vi "1st.vi"() -> ()   [LabVIEW 2016]
uses:
  <vilib>/Analysis/Matrix/Datatypes/RealMatrix.ctl
  <vilib>/Analysis/Matrix/Numeric/Conversions/Array To Matrix - RA.vi
  <vilib>/Analysis/Matrix/Numeric/Multiply/Multiply - RM,RM.vi
  <vilib>/Analysis/baseanly.llb/Real Inverse Matrix.vi
  <vilib>/Analysis/Matrix/Numeric/Conversions/Matrix To Array - RM.vi
  <vilib>/Analysis/Matrix/NI_Matrix.lvlib
  <vilib>/Analysis/NI_AALBase.lvlib
panel:
  out "r":dbl[](array[numeric])
  out "theta":dbl[](array[numeric])
  out "b":dbl[](array[numeric])
  out "a":dbl[](array[numeric])
  out "Real 2D Array":dbl[][](array[numeric])
  out "Final magnitude":T1
  in  "stop":bool
  out "Inverse Matrix":T1
  out "S(t)* X":T1
  in  "S":T1
  out "Matrix X":T1
  out "Array X":dbl[](array[numeric])
  in  "samples":dbl
  in  "Magnitude":dbl
  in  "Phase":dbl
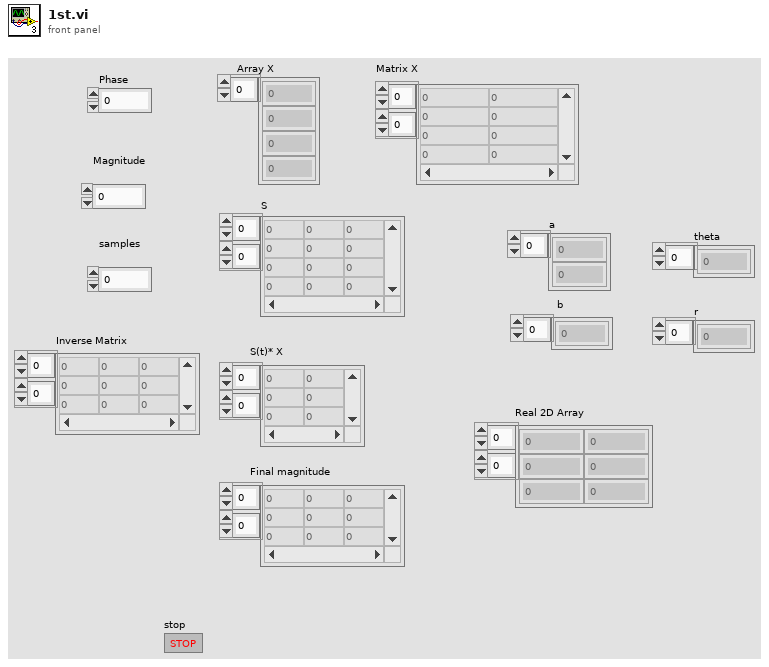
[diagram p1: front panel]
types:
  T1 = typedef "NI_Matrix.lvlib/RealMatrix.ctl" = dbl[][]
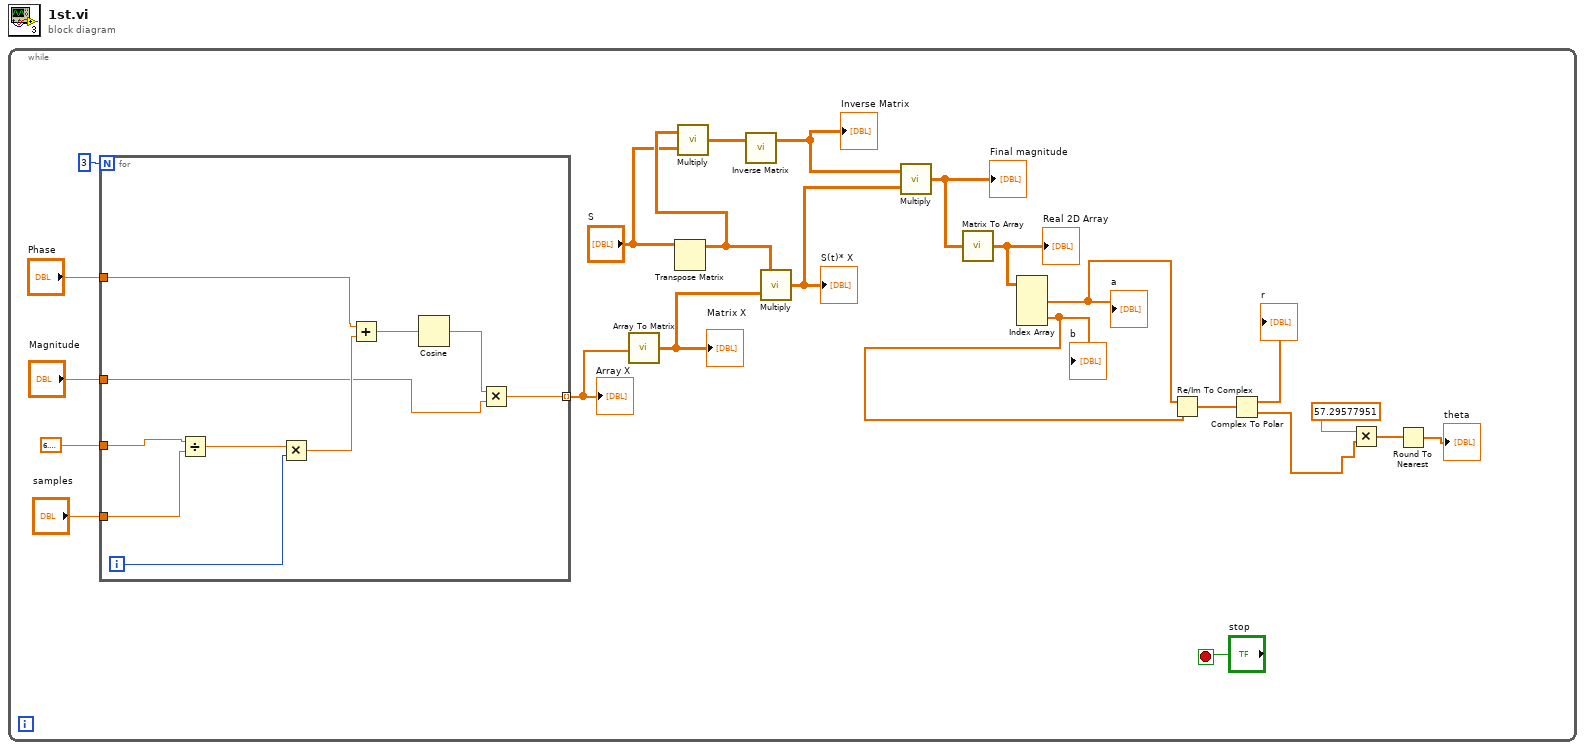
[diagram p0: block diagram]
diagram:
  n1 = while {
    stop <- "stop" stop-if-true
    n2 = for {
      N: 3 -> [_]
      tunnel: 6.283185307179586 -> [w33]
      tunnel: "samples" -> [w32]
      tunnel: "Phase" -> [w28]
      tunnel: "Magnitude" -> [w26]
      tunnel: [w25] -> w18 mode=indexing
      i -> [w30]
      n3 = Divide(x=w33, y=w32) -> (x/y=w31:dbl)
      n4 = Multiply(x=w31, y=w30) -> (x*y=w29:dbl)
      n5 = Add(x=w28, y=w29) -> (x+y=w27:dbl)
      n6 = Cosine(x=w27) -> (cos(x)=w24:dbl)
      n7 = Multiply(x=w24, y=w26) -> (x*y=w25:dbl)
    }
    "Array X" <- w18
    n8 = call-poly <vilib>:"Array To Matrix.vi"("Real 1D Array"=w18) -> ("Real Matrix (Column Vector)"=w17:T1)
    "Matrix X" <- w17
    n9 = Transpose Matrix(1:"S") -> (0:w14:T1)
    n10 = call-poly <vilib>:"Multiply.vi"("Real Matrix B"="S", "Real Matrix A"=w14) -> ("A * B"=w16:T1)
    n11 = call-poly <vilib>:"Inverse Matrix.vi"("Input Matrix"=w16) -> ("Inverse Matrix"=w13:T1)  [unwired: 1 in, 1 out]
    "Inverse Matrix" <- w13
    n12 = call-poly <vilib>:"Multiply.vi"("Real Matrix B"=w17, "Real Matrix A"=w14) -> ("A * B"=w12:T1)
    "S(t)* X" <- w12
    n13 = call-poly <vilib>:"Multiply.vi"("Real Matrix B"=w12, "Real Matrix A"=w13) -> ("A * B"=w11:T1)
    "Final magnitude" <- w11
    n14 = call-poly <vilib>:"Matrix To Array.vi"("Real Matrix"=w11) -> ("Real 2D Array"=w10:dbl[][])
    "Real 2D Array" <- w10
    n15 = Index Array(array=w10) -> (element #1=w9:dbl[], element #2=w8:dbl[])  [unwired: 4 in]
    "a" <- w9
    "b" <- w8
    n16 = Re/Im To Complex(1:w8, 2:w9) -> (0:w7:cdb[])
    n17 = Complex To Polar(r * e^(i*theta)=w7) -> (r=→"r":dbl[], theta=w4:dbl[])
    n18 = Multiply(x=57.29577951, y=w4) -> (x*y=w3:dbl[])
    n19 = Round To Nearest(number=w3) -> (nearest integer value=→"theta":dbl[])
  }
